vi "get_value.vi"(8 "error in (no error)":errorcluster, 10 "channel":dbl, 11 "Simulated_Instrument in":refnum<class "Simulated_Instrument.lvclass">) -> (0 "error out":errorcluster, 2 "value":string, 3 "Simulated_Instrument out":refnum<class "Simulated_Instrument.lvclass">)   [LabVIEW 2018, in "Simulated_Instrument.lvclass"]
doc: "the vi reads the value (pressure, temp etc etc) from the instrument.\nA radom number is returned."
uses:
  Simulated_Instrument.lvclass
  instrument.lvclass
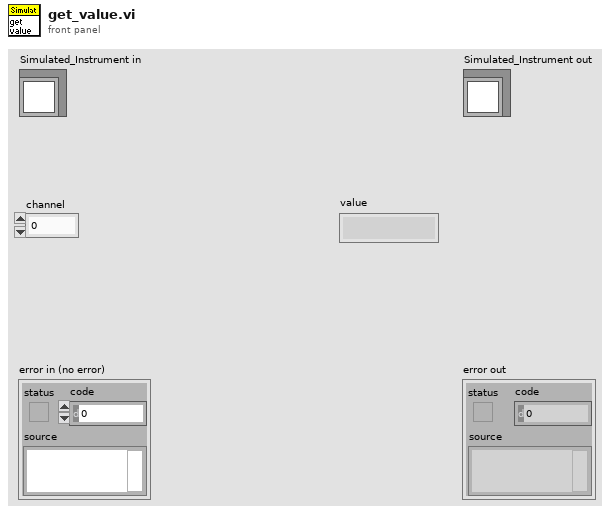
[diagram p1: front panel]
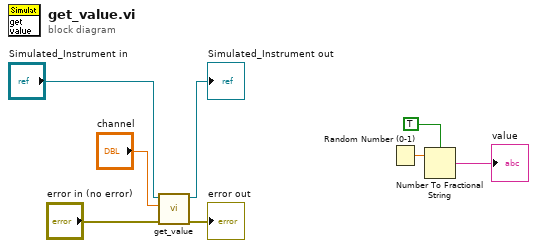
[diagram p0: block diagram]
diagram:
  n1 = call-parent "get_value.vi"("error in (no error)"="error in (no error)", "channel"="channel", "instrument in"="Simulated_Instrument in") -> ("error out"=→"error out":errorcluster, "instrument out"=→"Simulated_Instrument out":refnum<class "Simulated_Instrument.lvclass">)  [unwired: 6 in, 1 out]
  n2 = Random Number (0-1)() -> (number: 0 to 1=w3:dbl)
  n3 = Number To Fractional String(use system decimal point (T)=TRUE, number=w3) -> (F-format string=→"value":string)  [unwired: 2 in]
